vi "Send Last Ack.vi"(8 "error from actor":errorcluster, 9 "Caller-to-Actor Enqueuer":refnum<class "Message Enqueuer.lvclass">, 10 "Actor":refnum<class "Actor.lvclass">, 11 "Message Enqueuer":refnum<class "Message Enqueuer.lvclass">) -> ()   [LabVIEW 2017, in "Actor Framework.lvlib" / "Last Ack.lvclass"]
uses:
  <vilib>/ActorFramework/LastAck/Last Ack.lvclass
  <vilib>/ActorFramework/Actor/Actor.lvclass
  <vilib>/ActorFramework/Message Enqueuer/Message Enqueuer.lvclass
  e:/builds/penguin/labview/branches/2017/dev/dist/vi.lib/ActorFramework/Message/Message.lvclass
  <vilib>/ActorFramework/LastAck/Last Ack.lvclass/Last Ack.ctl
  <vilib>/ActorFramework/Message Enqueuer/Message Enqueuer.lvclass/Message Enqueuer.ctl
  <vilib>/ActorFramework/Message Priority Queue/Priority Enqueue.vi
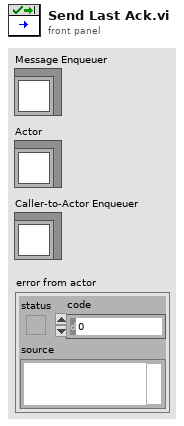
[diagram p1: front panel]
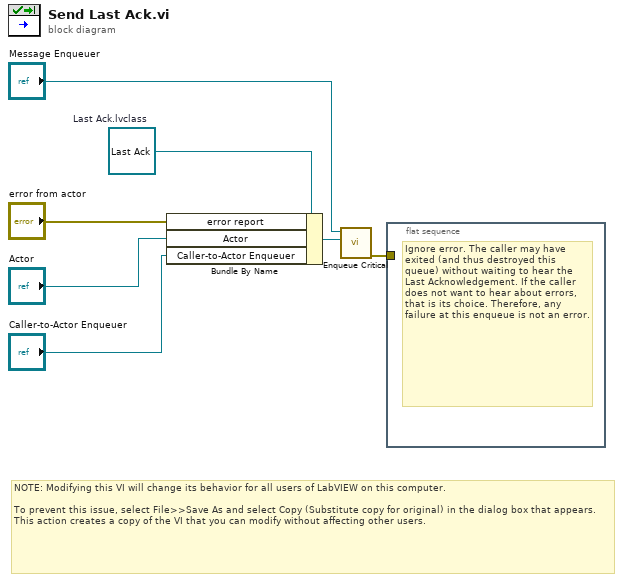
[diagram p0: block diagram]
diagram:
  w7 = refnum<class "Last Ack.lvclass"> refnum  # Last Ack.lvclass
  # "NOTE: Modifying this VI will change its behavior for all users of LabVIEW on this computer.\n\nTo prevent this issue, select File>>Save As and select Copy (Substitute copy for original) in the dialog box that appears. This action creates a copy of the VI that you can modify without affecting other users."
  n1 = Bundle By Name(cluster=w7, "error report"="error from actor", "Actor"="Actor", "Caller-to-Actor Enqueuer"="Caller-to-Actor Enqueuer") -> (w2:refnum<class "Last Ack.lvclass">)
  n2 = call <vilib>:"Enqueue Critical.vi"("Message"=w2, "Message Enqueuer in"="Message Enqueuer") -> ("error out"=w1:errorcluster)  [unwired: 8 in, 1 out]
  n3 = flat-sequence {
    tunnel: w1 -> [_]
    frame #0 {
      # "Ignore error. The caller may have exited (and thus destroyed this queue) without waiting to hear the Last Acknowledgement. If the caller does not want to hear about errors, that is its choice. Therefore, any failure at this enqueue is not an error."
    }
  }
